vi "Year2016_Question1.vi"() -> ()   [LabVIEW 2015]
panel:
  in  "c":dbl
  in  "b":dbl
  in  "a":dbl
  out "Alpha in degrees":dbl
  in  "stop":bool
  out "Alpha in radian":dbl
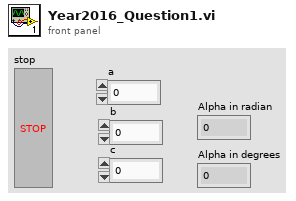
[diagram p1: front panel]
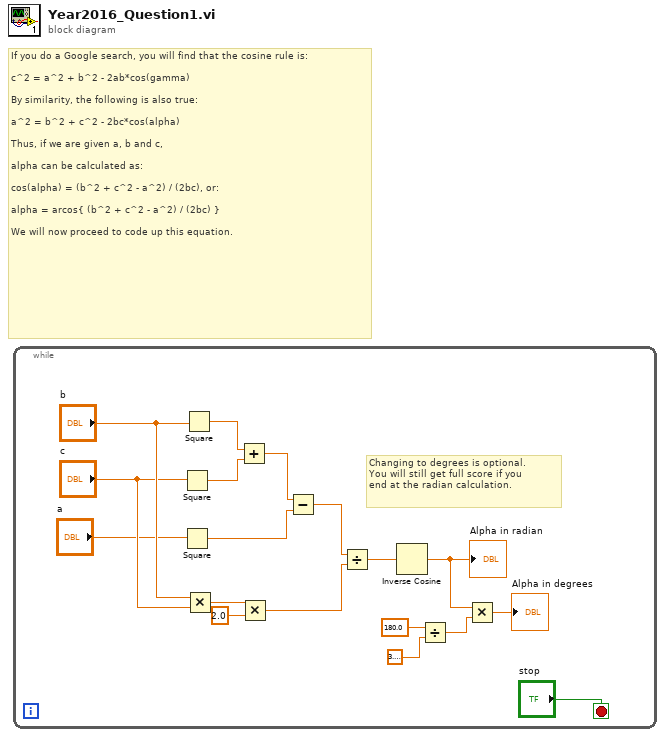
[diagram p0: block diagram]
diagram:
  # "If you do a Google search, you will find that the cosine rule is:\n\nc^2 = a^2 + b^2 - 2ab*cos(gamma)\n\nBy similarity, the following is also true:\n\na^2 = b^2 + c^2 - 2bc*cos(alpha)\n\nThus, if we are given a, b and c, \n\nalpha can be calculated as:\n\ncos(alpha) = (b^2 + c^2 - a^2) / (2bc), or:\n\nalpha = arcos{ (b^2 + c^2 - a^2) / (2bc) }\n\nWe will now proceed to code up this equation."
  n1 = while {
    stop <- "stop" stop-if-true
    # "Changing to degrees is optional.\nYou will still get full score if you\nend at the radian calculation."
    n2 = Square(x="c") -> (x^2=w17:dbl)
    n3 = Square(x="a") -> (x^2=w15:dbl)
    n4 = Square(x="b") -> (x^2=w18:dbl)
    n5 = Multiply(x="b", y="c") -> (x*y=w14:dbl)
    n6 = Add(x=w18, y=w17) -> (x+y=w16:dbl)
    n7 = Multiply(x=w14, y=2.0) -> (x*y=w11:dbl)
    n8 = Subtract(x=w16, y=w15) -> (x-y=w12:dbl)
    n9 = Divide(x=w12, y=w11) -> (x/y=w10:dbl)
    n10 = Inverse Cosine(1:w10) -> (0:w8:dbl)
    "Alpha in radian" <- w8
    n11 = Divide(x=180.0, y=3.141592653589793) -> (x/y=w7:dbl)
    n12 = Multiply(x=w8, y=w7) -> (x*y=→"Alpha in degrees":dbl)
  }
